vi "FIFO Publisher Return Command.vi"(8 "error in":errorcluster, 10 "FIFO Publisher":T1, 11 "ChanMngOOB_Tx in":refnum<class "ChnMngOOB_Tx.lvclass">) -> (0 "error out":errorcluster, 3 "ChanMngOOB_Tx out":refnum<class "ChnMngOOB_Tx.lvclass">)   [LabVIEW 2021, in "ChnMngOOB_Tx.lvclass"]
uses:
  ChnMngOOB_Tx.lvclass
  C:/Program Files/National Instruments/LabVIEW 2021/vi.lib/CIF Foundation/CIF Out of Band Commands/CIFOutOfBand.lvclass
  Typedef/FIFO Publisher Return.ctl
  <vilib>/CIF Foundation/CIF Out of Band Commands/CIFOutOfBand.lvclass/CIFOutOfBand.ctl
  <vilib>/CIF Foundation/CIF Out of Band Commands/Typedef/OOB Container.ctl
  Typedef/Template Payload.ctl
  typedef/Channel List for OOB.ctl
  <vilib>/CIF Foundation/CIF Channels Core/CIFChannels/Typedef/Direction.ctl
  Typedef/OOB Core Commands.ctl
  <vilib>/CIF Foundation/CIF Out of Band Commands/CIFOutOfBand.lvclass
  <vilib>/CIF Foundation/CIF Channels Core/CIFChannels/CIFChannels.lvclass
  CIFChannelMng.lvclass
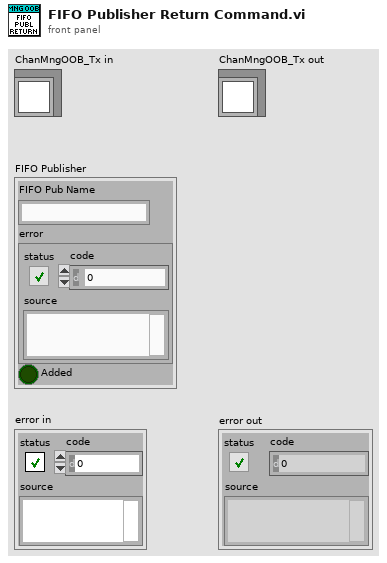
[diagram p1: front panel]
types:
  T1 = typedef "ChnMngOOB_Tx.lvclass/FIFO Publisher Return.ctl" = cluster{"FIFO Pub Name":string, "error":errorcluster, "Added":bool}
  T2 = typedef "CIFOutOfBand.lvclass/OOB Container.ctl" = cluster{"Commands (bitwise)":u64, "Payload":variant}
  T3 = typedef "ChnMngOOB_Tx.lvclass/Template Payload.ctl" = cluster{"Channel List":T4[], "New FIFO Publisher":T1}
  T4 = typedef "CIFChannelMng.lvclass/Channel List for OOB.ctl" = cluster{"Name":string, "Direction":T5, "Type":string, "Connected?":bool, "Connected Name":string, "Custom Config Data":u8[], "Forced?":bool}
  T5 = typedef "CIFChannels.lvclass/Direction.ctl" = enum16{"Publisher", "Subscriber"}
  T6 = typedef "ChnMngOOB_Tx.lvclass/OOB Core Commands.ctl" = enum8{"Channel List", "New FIFO Pub"}
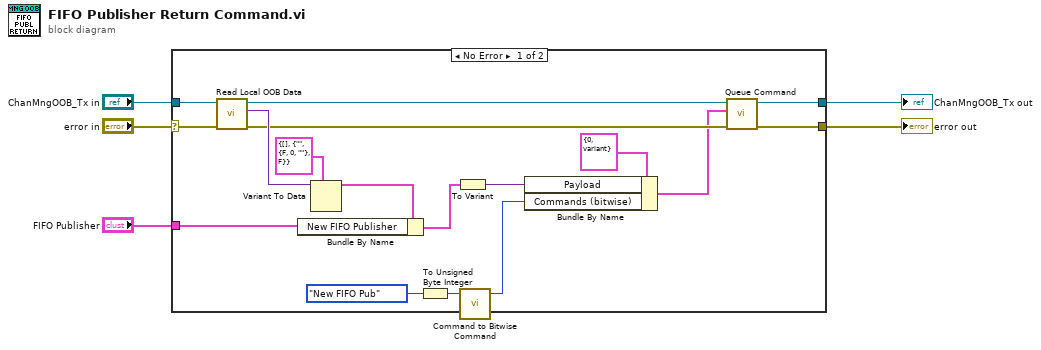
[diagram p0: block diagram]
diagram:
  n1 = case shown="No Error" "error in" {
    selector: "error in" -> [w20 w24]
    tunnel: [w21 w24] -> w4
    tunnel: "ChanMngOOB_Tx in" -> [w19 w23]
    tunnel: [w22 w23] -> w2
    tunnel: "FIFO Publisher" -> [w6 _]
    frame No Error {
      n2 = call <vilib>:"Read Local OOB Data.vi"("error in"=w20, "OOB in"=w19) -> ("error out"=w10:errorcluster, "Local OOB Data"=w14:variant, "OOB out"=w9:refnum<class "ChnMngOOB_Tx.lvclass">)  [unwired: 7 in]
      n3 = Variant To Data(type=T3 {"Channel List"=[], "New FIFO Publisher"={"FIFO Pub Name"="", "error"={"status"=FALSE, "code"=0, "source"=""}, "Added"=FALSE}} ("Template Payload"), Variant=w14) -> (data=w16:T3)  [unwired: 1 in, 1 out]
      n4 = Bundle By Name(cluster=w16, "New FIFO Publisher"=w6) -> (w15:T3)
      n5 = To Unsigned Byte Integer(number=OOB_Core_Commands."New FIFO Pub" ("OOB Main Commands")) -> (unsigned 8bit integer=w18:u8)
      n6 = To Variant(anything=w15) -> (Variant=w11:variant)
      n7 = call <vilib>:"Command to Bitwise Command.vi"("Command"=w18) -> ("bit command"=w8:u64)  [unwired: 3 in]
      n8 = Bundle By Name(cluster=T2 {"Commands (bitwise)"=0, "Payload"=variant} ("OOB Data"), "Payload"=w11, "Commands (bitwise)"=w8) -> (w7:T2)
      n9 = call <vilib>:"Queue Command.vi"("error in"=w10, "OOB Data"=w7, "OOB in"=w9) -> ("error out"=w21:errorcluster, "OOB out"=w22:refnum<class "ChnMngOOB_Tx.lvclass">)  [unwired: 7 in]
    }
    frame Error {
    }
  }
  "error out" <- w4
  "ChanMngOOB_Tx out" <- w2
